vi "Create and Add Instruments.vi"(7 "Is Target?":bool, 8 "Error In":errorcluster, 10 "Instr CFGs":string[](array[string]), 11 "MSS in":refnum<class "MSS.lvclass">) -> (0 "Error Out":errorcluster, 2 "Target Instr CFGs":string[](array[string]), 3 "MSS out":refnum<class "MSS.lvclass">)   [LabVIEW 2024, in "HAL.lvlib" / "MSS.lvclass"]
uses:
  MSS.lvclass
  Configurations/CFG JSON/CFG JSON.lvclass
  25b25780-789a-4bec-9ea7-0fafa89e9659.vi
  444cf0ba-9258-4d70-83a7-5f5fa0944b3f.vi
  25b25780-789a-4bec-9ea7-0fafa89e9659.vi/a4169a97-72fc-4003-a778-603cf20cafa0.vi
  444cf0ba-9258-4d70-83a7-5f5fa0944b3f.vi/a4169a97-72fc-4003-a778-603cf20cafa0.vi
  <vilib>/JDP Science/JSONtext/Find Item.vi
  <vilib>/JDP Science/JSONtext/Next JSON Value.vi
  <vilib>/JDP Science/JSONtext/String Subset.vi
  <vilib>/JDP Science/JSONtext/Parsing/Advance past next JSON Value (inlined COPY).vi
  <vilib>/JDP Science/JSONtext/Parsing/Advance past whitespace.vi
  <vilib>/JDP Science/JSONtext/Parsing/Advance past String.vi
  <vilib>/JDP Science/JSONtext/Parsing/Advance past Number.vi
  <vilib>/JDP Science/JSONtext/Parsing/Advance past Line Ending.vi
  <vilib>/JDP Science/JSONtext/Parsing/Parse Full Path or Item Name.vi
  <vilib>/JDP Science/JSONtext/Parsing/Advance past Array.vi
  <vilib>/JDP Science/JSONtext/Parsing/Advance past Object.vi
  <vilib>/JDP Science/JSONtext/support/Error Cluster From Code.vi
  <vilib>/JDP Science/JSONtext/Offset/Find Item Locations by Path.vi
  <vilib>/JDP Science/JSONtext/JSON text to Variant.vi
  <vilib>/Utility/error.llb/Error Cluster From Error Code.vi
  <vilib>/JDP Science/JSONtext/LVClass Serializer/JSONtext LVClass Serializer.lvclass
  Instrument/Instrument.lvclass
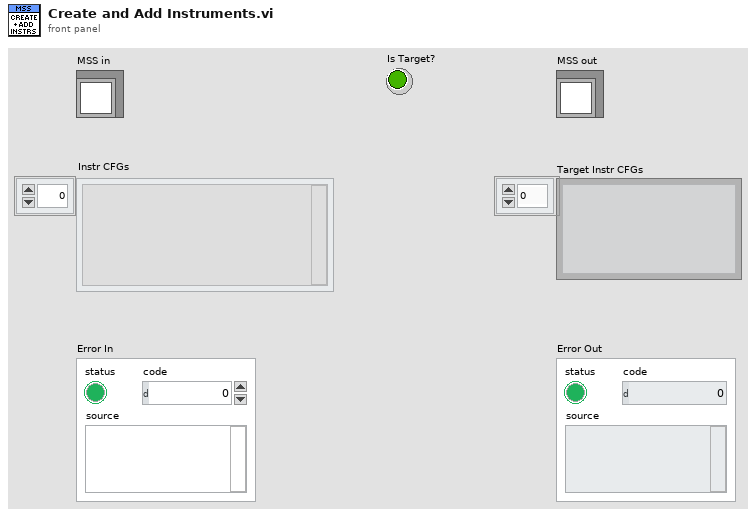
[diagram p1: front panel]
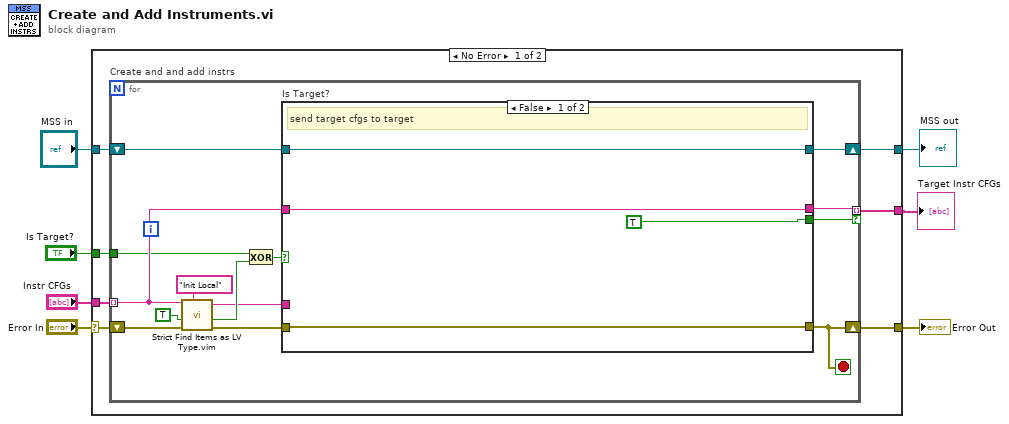
[diagram p0: block diagram]
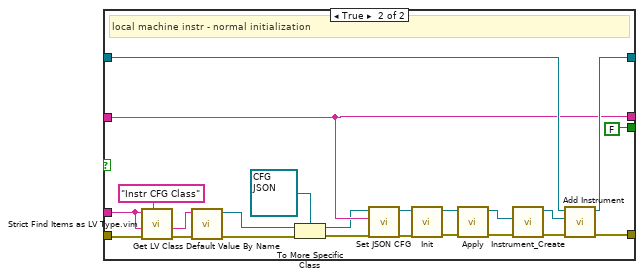
[diagram p2: hidden frame]
diagram:
  n1 = case shown="No Error" "Error In" {
    selector: "Error In" -> [w12 w55]
    tunnel: [w10 w55] -> w7
    tunnel: [w13 w56] -> w3
    tunnel: "MSS in" -> [w14 w56]
    tunnel: "Instr CFGs" -> [w11 _]
    tunnel: [w9 _] -> w2
    tunnel: "Is Target?" -> [w8 _]
    frame No Error {
      n2 = for "Create and and add instrs" {
        shift-right: [w24] -> w10
        shift-left: w12 -> [w28]
        tunnel: w11 -> [w21] mode=indexing
        shift-right: [w27] -> w13
        shift-left: w14 -> [w26]
        tunnel: [w25] -> w9 mode=indexing if=w23
        tunnel: w8 -> [w16]
        stop <- w24 stop-if-true
        n3 = call "Strict Find Items as LV Type.vim"("$Path or Item Name"="Init Local", "error in"=w28, "Data Type and Default Value"=TRUE, "<JSON>"=w21) -> ("error out"=w20:errorcluster, "Data out"=w17:bool, "<JSON> duplicate"=w15:string)  [unwired: 5 in]
        n4 = Exclusive Or(1:w17, 2:w16) -> (0:w22:bool)
        n5 = case "Is Target?" shown="False" w22 {
          tunnel: [w31 w48] -> w24
          tunnel: w26 -> [w32 w47]
          tunnel: [w32 w46] -> w27
          tunnel: w20 -> [w31 w42]
          tunnel: w21 -> [w30 w45]
          tunnel: [w30 w45] -> w25
          tunnel: [TRUE FALSE] -> w23
          tunnel: w15 -> [_ w33]
          frame False {
            # "send target cfgs to target"
          }
          frame True {
            # "local machine instr - normal initialization"
            n6 = call "Strict Find Items as LV Type.vim"("$Path or Item Name"="Instr CFG Class", "error in"=w42, "Data Type and Default Value"=w33, "<JSON>"=w33) -> ("error out"=w43:errorcluster, "Data out"=w34:string)  [unwired: 5 in, 1 out]
            n7 = call <vilib>:"Get LV Class Default Value By Name.vi"("error in (no error)"=w43, "class name"=w34) -> ("error out"=w40:errorcluster, "object"=w39:refnum<class>)  [unwired: 8 in]
            n8 = To More Specific Class(target class=refnum<class "CFG JSON.lvclass"> refnum ("HAL.lvlib:CFG JSON.lvclass"), reference=w39, error in=w40) -> (specific class reference=w37:refnum<class "CFG JSON.lvclass">, error out=w36:errorcluster)
            n9 = call "Set JSON CFG.vi"("<JSON> CFG"=w45, "CFG JSON in"=w37) -> ("CFG JSON out"=w52:refnum<class "CFG JSON.lvclass">)  [unwired: 9 in]
            n10 = call-dynamic "Init.vi"("error in"=w36, "CFG Base in"=w52) -> ("error out"=w53:errorcluster, "CFG Base out"=w50:refnum<class "CFG JSON.lvclass">)  [unwired: 8 in]
            n11 = call-dynamic "Apply.vi"("error in"=w53, "CFG Base in"=w50) -> ("error out"=w51:errorcluster, "CFG Base out"=w35:refnum<class "CFG JSON.lvclass">)  [unwired: 8 in]
            n12 = call "Instrument_Create.vi"("Error In"=w51, "CFG Base"=w35) -> ("Error Out"=w54:errorcluster, "reference out"=w49:refnum<class "Instrument.lvclass">)  [unwired: 8 in]
            n13 = call "Add Instrument.vi"("error in"=w54, "Instrument"=w49, "MSS in"=w47) -> ("error out"=w48:errorcluster, "MSS out"=w46:refnum<class "MSS.lvclass">)  [unwired: 7 in]
          }
        }
      }
    }
    frame Error {
    }
  }
  "MSS out" <- w3
  "Error Out" <- w7
  "Target Instr CFGs" <- w2
